vi "main_120MHz.vi"() -> ()   [LabVIEW 2010]
uses:
  common_typedefs/channels_cluster.ctl
  common_typedefs/gate_parameters_cluster.ctl
  common_typedefs/pixel_to_host_enum.ctl
  <vilib>/Platform/TimedLoop/XDataNode/XDataNode.xnode
  <vilib>/Platform/TimedLoop/XDataNode/timing_clust.ctl
  <vilib>/Platform/TimedLoop/XDataNode/nitl_modes.ctl
  <vilib>/Platform/TimedLoop/XDataNode/wakeup.ctl
  <vilib>/eio/EIONode/EIONode.xnode
  <vilib>/rvi/eio/nirviEIOImplementation/nirviEIOImplementation.xnode
  <vilib>/rvi/eio/common/nirviEmuClasses.ctl
  <vilib>/rvi/eio/common/nirviEmuTemplateMethod_noerrors.vi
  <vilib>/Platform/TimedLoop/XDataNode/XDNodeRunTimeDep.lvlib
panel:
  in  "pixel-to-host mode":T1
  in  "gate 3":T2
  in  "gate 2":T2
  in  "gate 1":T2
  out "integrated pixel values":T3
  out "data read":T3
  in  "channel offsets":T3
  out "clock 3 state":bool
  out "clock 2 state":bool
  out "clock 1 state":bool
  in  "stop acquisition at FIFO overflow?":bool=TRUE
  in  "wait for trigger?":bool
  in  "stop":bool
  in  "acquire":bool
  out "acquiring?":bool
  out "FIFO overflow":bool
  out "current pixel no.":i64
  in  "number of pixels":i64=-1
  in  "maximum bit depth":i8
  in  "iterations per pixel":u32
  in  "enable ADC clock?":bool=TRUE
  in  "ADC clock phase":u8
  in  "converter box version":i16=1 min=1 max=2
  # "Outputs / displays"
  # "Integration parameters"
  # "Clock parameters"
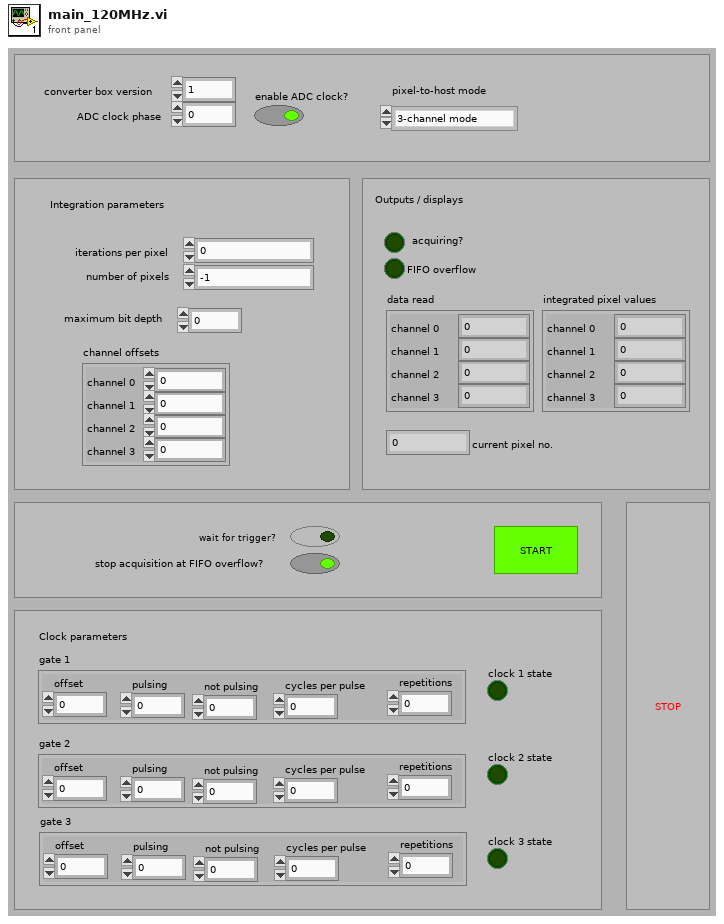
[diagram p1: front panel]
types:
  T1 = typedef "pixel_to_host_enum.ctl" = enum16{"3-channel mode", "4-channel mode"}
  T2 = typedef "gate_parameters_cluster.ctl" = cluster{"offset":i64, "pulsing":i64, "not pulsing":i64, "cycles per pulse":i64, "repetitions":i64}
  T3 = typedef "channels_cluster.ctl" = cluster{"channel 0":u32, "channel 1":u32, "channel 2":u32, "channel 3":u32}
  T4 = typedef "XDNodeRunTimeDep.lvlib/timing_clust.ctl" = cluster{"Expected End [f-1]":u64, "Actual End [f-1]":u64, "Finished Late? [f-1]":bool, "Expected End [i-1]":u64, "Actual End [i-1]":u64, "Finished Late? [i-1]":bool, "Expected Start [i]":u64, "Actual Start [i]":u64, "Expected Start [f]":u64, "Actual Start [f]":u64, "Source Name":string, "Structure Name":string, "Period":i64, "Deadline":i64, "Offset":i64, "Start":i64, "Priority":i32, "Timeout":i32, "Mode":T5, "Wakeup Reason":T6, "Error":errorcluster, "Source Type":string, "Secondary Source Type":string, "Global End Time":u64, "Global Start Time":u64, "Frame Duration":u64, "Iteration Duration":u64, "Assigned CPU":i32, "I/O Scan Engine Mode":u32}
  T5 = typedef "XDNodeRunTimeDep.lvlib/nitl_modes.ctl" = enum32{"No Change", "Process missed periods, maintain original phase", "Discard missed periods, maintain original phase", "Process missed periods, ignore original phase", "Discard missed periods, ignore original phase"}
  T6 = typedef "XDNodeRunTimeDep.lvlib/wakeup.ctl" = enum32{"Normal", "Aborted", "Asynchronous wakeup", "Timing source error", "Timed loop error", "Timeout"}
  T7 = typedef "nirviEmuClasses.ctl" = enum16{"IO Read", "IO Write", "Method", "Property Read", "Property Write"}
  T8 = typedef "gate_counters_cluster.ctl" = cluster{"phase iteration counter":i64, "phase repetition counter":i64, "pulse iteration counter":i64, "phase state":bool}
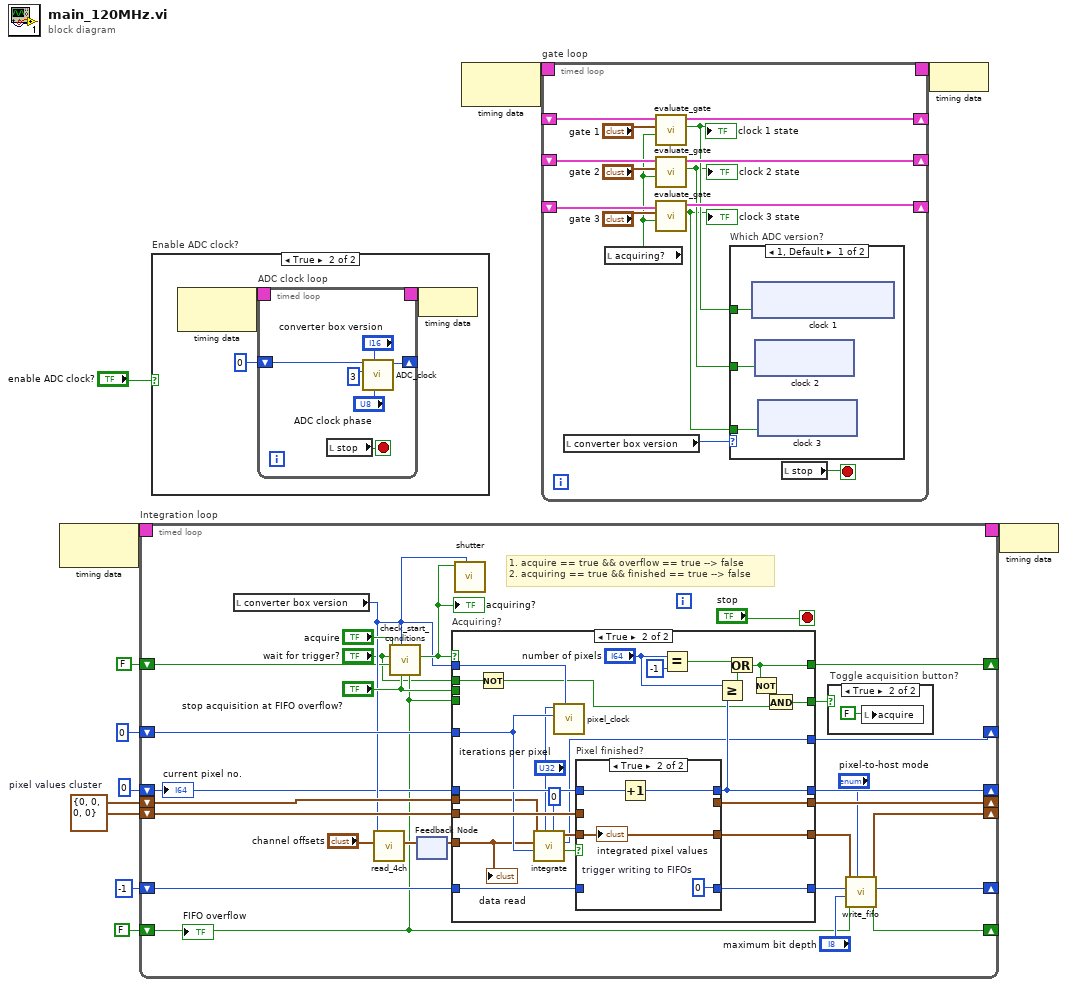
[diagram p0: block diagram]
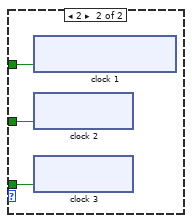
[diagram p2: hidden frame]
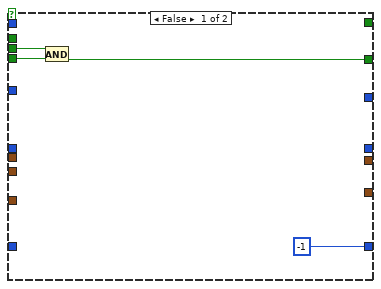
[diagram p4: hidden frame]
diagram:
  w4 = T3 {"channel 0"=0, "channel 1"=0, "channel 2"=0, "channel 3"=0}  # pixel values cluster
  n1 = node-c288() -> (w10:T4)  [unwired: 1 in]
  n2 = timed-loop "Integration loop" {
    timing: w10 -> [_]
    timing-out: [_] -> w9
    shift-right: [w32] -> _
    shift-left: i64 0 -> [w17]
    shift-right: [w31] -> _
    shift-left: u32 0 ("iteration counter out") -> [w35]
    shift-right: [w33] -> _
    shift-left: w4 -> [w37]
    shift-right: [w18] -> _
    shift-left: FALSE -> [w14]
    shift-right: [w23] -> _
    shift-left: w4 -> [w34]
    shift-right: [w20] -> _
    shift-left: -1 ("block index out") -> [w36]
    shift-right: [w26] -> _
    shift-left: FALSE -> [w15]
    stop <- "stop" stop-if-true
    # "1. acquire == true && overflow == true --> false\n2. acquiring == true && finished == true --> false"
    n3 = local read "converter box version"() -> (w24:i16)
    n4 = call "read_4ch.vi"("channel offsets"="channel offsets", "converter box version"=w24) -> ("read output"=w29:T3)  [unwired: 9 in]
    n5 = call "check_start_conditions.vi"("FIFO overflow?"=w14, "stop at FIFO overflow?"="stop acquisition at FIFO overflow?", "converter box version"=w24, "already acquiring?"=w15, "in triggered mode?"="wait for trigger?", "acquire"="acquire") -> ("acquire?"=w25:bool)  [unwired: 5 in]
    "acquiring?" <- w25
    n6 = feedback-in #1(w29) -> ()
    n7 = feedback #1() -> (w28:T3)  [unwired: 1 in]
    n8 = case "Acquiring?" shown="True" w25 {
      tunnel: w24 -> [_ w69]
      tunnel: [_ w51] -> w22
      tunnel: [_ w59] -> w31
      tunnel: [_ w65] -> w32
      tunnel: w37 -> [_ w56]
      tunnel: w36 -> [_ w54]
      tunnel: w17 -> [_ w63]
      tunnel: w35 -> [_ w58]
      tunnel: w34 -> [_ w62]
      tunnel: [_ w64] -> w33
      tunnel: [-1 ("block index out") w52] -> w19
      tunnel: w28 -> [_ w57]
      tunnel: "stop acquisition at FIFO overflow?" -> [w43 _]
      tunnel: [_ w49] -> w26
      tunnel: [w41 w46] -> w12
      tunnel: w14 -> [w42 _]
      tunnel: "wait for trigger?" -> [_ w48]
      frame False {
        n9 = And(x=w42, y=w43) -> (x .and. y?=w41:bool)
      }
      frame True {
        n10 = Not(x=w48) -> (.not. x?=w45:bool)
        n11 = call "integrate.vi"("waiting iterations per pixel"=u32 0, "integration iterations per pixel"="iterations per pixel", "iteration counter in"=w58, "sampling values in"=w57, "previous pixel values in"=w56) -> ("finished?"=w61:bool, "iteration counter out"=w59:u32, "new pixel values out"=w60:T3)  [unwired: 4 in]
        n12 = call "pixel_clock.vi"("converter box version"=w69, "current iteration"=w58, "iterations per pixel"="iterations per pixel") -> ()  [unwired: 9 in]
        n13 = case "Pixel finished?" shown="True" w61 {
          tunnel: w60 -> [w73 w77]
          tunnel: [w72 w77] -> w51
          tunnel: [w71 w75] -> w65
          tunnel: w63 -> [w71 w76]
          tunnel: [w73 _] -> w64
          tunnel: w62 -> [w72 _]
          tunnel: w54 -> [w70 _]
          tunnel: [w70 w74] -> w52
          frame False {
          }
          frame True {
            w74 = 0  # trigger writing to FIFOs
            n14 = Increment(x=w76) -> (x+1=w75:i64)
            "integrated pixel values" <- w77
          }
        }
        n15 = Equal?(x="number of pixels", y=i64 -1 ("x")) -> (x = y?=w68:bool)
        n16 = Greater Or Equal?(x="number of pixels", y=w65) -> (x >= y?=w67:bool)
        n17 = Or(x=w68, y=w67) -> (x .or. y?=w49:bool)
        n18 = Not(x=w49) -> (.not. x?=w47:bool)
        n19 = And(x=w47, y=w45) -> (x .and. y?=w46:bool)
        "data read" <- w57
      }
    }
    n20 = call "shutter.vi"("converter box version"=w24, "open?"=w25) -> ()  [unwired: 10 in]
    n21 = case "Toggle acquisition button?" shown="True" w12 {
      frame False {
      }
      frame True {
        n22 = local write "acquire"(FALSE) -> ()
      }
    }
    n23 = call "write_fifo.vi"("pixel-to-host\n mode"="pixel-to-host mode", "FIFO overflow in"=w14, "maximum bit depth"="maximum bit depth", "block index in"=w19, "values to be written"=w22) -> ("FIFO overflow out"=w18:bool, "block index out"=w20:i32, "channels out"=w23:T3)  [unwired: 4 in]
    "current pixel no." <- w17
    "FIFO overflow" <- w14
  }
  n24 = case "Enable ADC clock?" shown="True" "enable ADC clock?" {
    frame False {
    }
    frame True {
      n25 = node-c288() -> (w82:T4)  [unwired: 1 in]
      n26 = timed-loop "ADC clock loop" {
        timing: w82 -> [_]
        timing-out: [_] -> w81
        shift-right: [w87] -> _
        shift-left: u8 0 ("counter out") -> [w88]
        stop <- w84 stop-if-true
        n27 = local read "stop"() -> (w84:bool)
        n28 = call "ADC_clock.vi"("phase"="ADC clock phase", "converter box version"="converter box version", "iterations per cycle"=u8 3, "counter in"=w88) -> ("counter out"=w87:u8)  [unwired: 7 in]
      }
      n29 = node-c288(w81) -> ()
    }
  }
  n30 = node-c288() -> (w3:T4)  [unwired: 1 in]
  n31 = timed-loop "gate loop" {
    timing: w3 -> [_]
    timing-out: [_] -> w2
    shift-right: [w106] -> _
    shift-left: _ -> [w107]
    shift-right: [w104] -> _
    shift-left: _ -> [w105]
    shift-right: [w103] -> _
    shift-left: _ -> [w102]
    stop <- w97 stop-if-true
    n32 = local read "converter box version"() -> (w96:i16)
    n33 = local read "acquiring?"() -> (w98:bool)
    n34 = call "evaluate_gate.vi"("acquiring?"=w98, "gate settings"="gate 1", "gate counters in"=w107) -> ("pulse state out"=w95:bool, "gate counters out"=w106:T8)  [unwired: 7 in]
    "clock 1 state" <- w95
    n35 = call "evaluate_gate.vi"("acquiring?"=w98, "gate settings"="gate 2", "gate counters in"=w105) -> ("pulse state out"=w94:bool, "gate counters out"=w104:T8)  [unwired: 7 in]
    "clock 2 state" <- w94
    n36 = call "evaluate_gate.vi"("acquiring?"=w98, "gate settings"="gate 3", "gate counters in"=w102) -> ("pulse state out"=w93:bool, "gate counters out"=w103:T8)  [unwired: 7 in]
    "clock 3 state" <- w93
    n37 = case "Which ADC version?" shown="1, Default" w96 {
      tunnel: w95 -> [w108 w146]
      tunnel: w94 -> [w109 w145]
      tunnel: w93 -> [w110 w144]
      frame 1, Default {
        n38 = xnode "clock 1"("Connector1/DIO32"=w108) -> ()  [unwired: 1 in, 1 out]
        n39 = xnode "clock 2"("PXI_RTSI_1"=w109) -> ()  [unwired: 1 in, 1 out]
        n40 = xnode "clock 3"("PXI_RTSI_2"=w110) -> ()  [unwired: 1 in, 1 out]
      }
      frame 2 {
        n41 = xnode "clock 1"("Connector0/DIO38"=w146) -> ()  [unwired: 1 in, 1 out]
        n42 = xnode "clock 2"("PXI_RTSI_1"=w145) -> ()  [unwired: 1 in, 1 out]
        n43 = xnode "clock 3"("PXI_RTSI_2"=w144) -> ()  [unwired: 1 in, 1 out]
      }
    }
    n44 = local read "stop"() -> (w97:bool)
  }
  n45 = node-c288(w2) -> ()
  n46 = node-c288(w9) -> ()
